vi "최치원저격용.vi"() -> ()   [LabVIEW 2015]
uses:
  <vilib>/NXT/Block Support/NXT_OutputPort.ctl
  <vilib>/NXT/Block Support/NXT_InputPort.ctl
  <vilib>/NXT/Subs/MotorOutput.ctl
  <vilib>/NXT/NXTIO Xnodes/NXTIONodeSubVIs/NXTMoveMotors.vi
  <vilib>/NXT/Dual Mode Library/Waits/Wait_Num.vi
  <vilib>/NXT/Dual Mode Library/Sensors/Sonar_cm.vi
  <vilib>/NXT/Dual Mode Library/Motors/MotorOn.vi
  <vilib>/NXT/Dual Mode Library/Waits/Wait_Rotation.vi
  <vilib>/NXT/Dual Mode Library/Sensors/Light_On.vi
  <vilib>/NXT/Dual Mode Library/Motors/MotorReverse.vi
  <vilib>/NXT/NXTIO Xnodes/AddressXNode/NXTIOAddress.xnode
  <vilib>/NXT/Subs/LVHSConnector.ctl
  <vilib>/NXT/NXTIO Xnodes/NXTIOXNode/NXTIO.xnode
  <vilib>/NXT/LegoClasses/BrickReference/BrickReference.lvclass
panel:
  in  "직진속도":i8=75
  in  "정지":bool
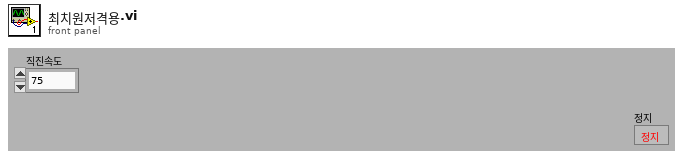
[diagram p1: front panel]
types:
  T1 = typedef "NXT_OutputPort.ctl" = u8
  T2 = typedef "LVHSConnector.ctl" = refnum<class "BrickReference.lvclass">
  T3 = typedef "MotorOutput.ctl" = u8
  T4 = typedef "NXT_InputPort.ctl" = u32
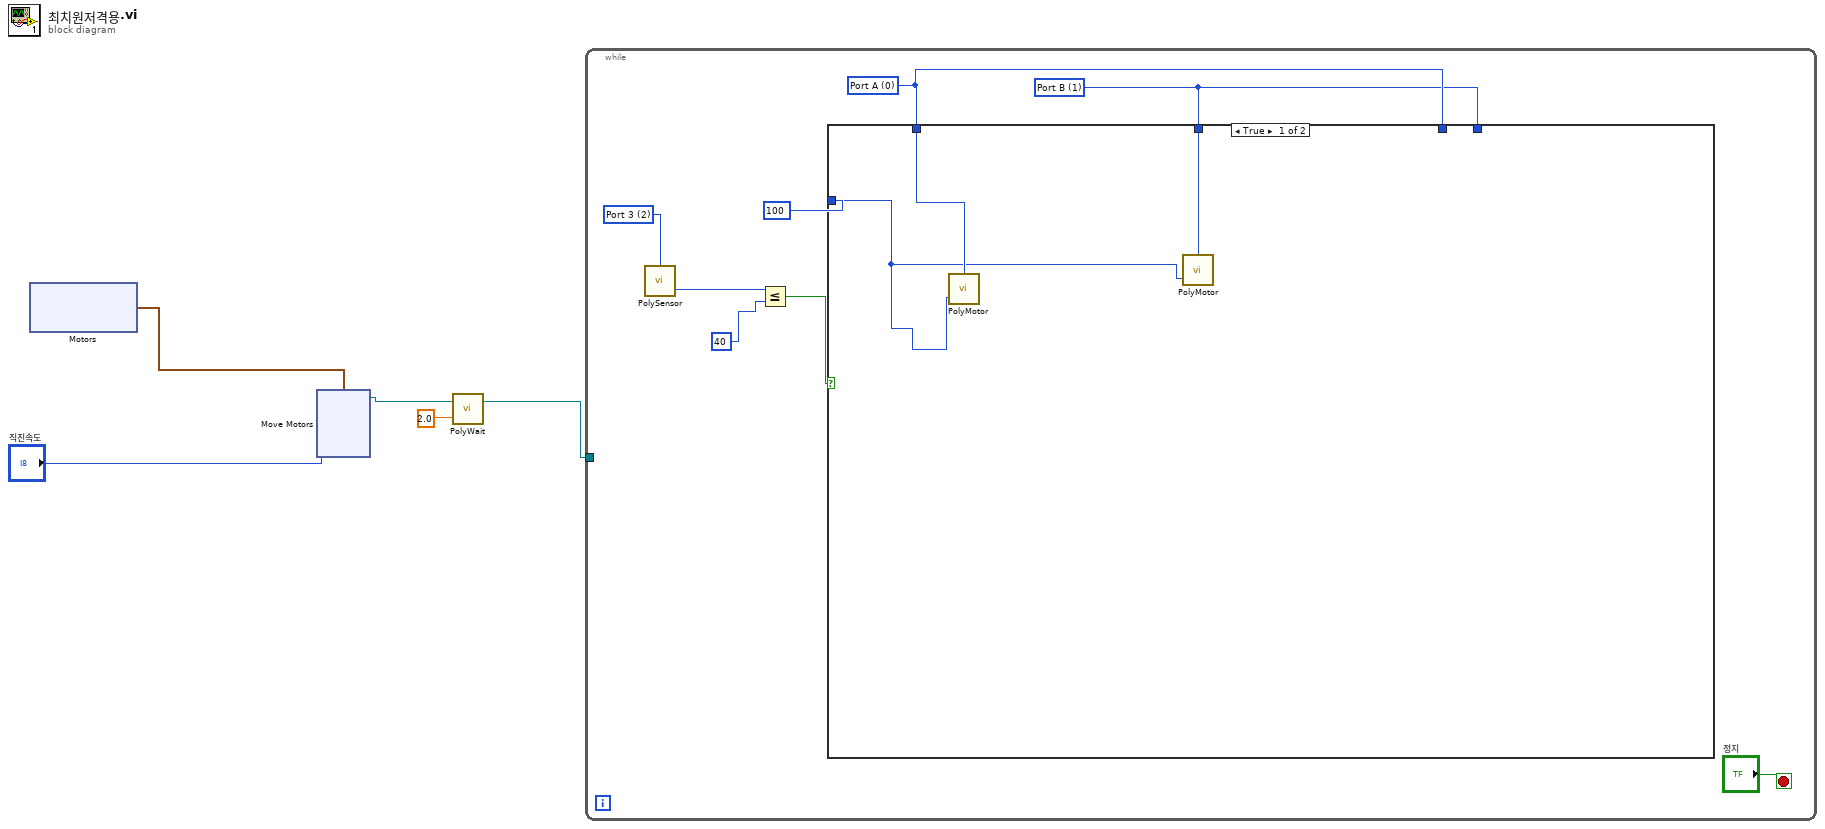
[diagram p0: block diagram]
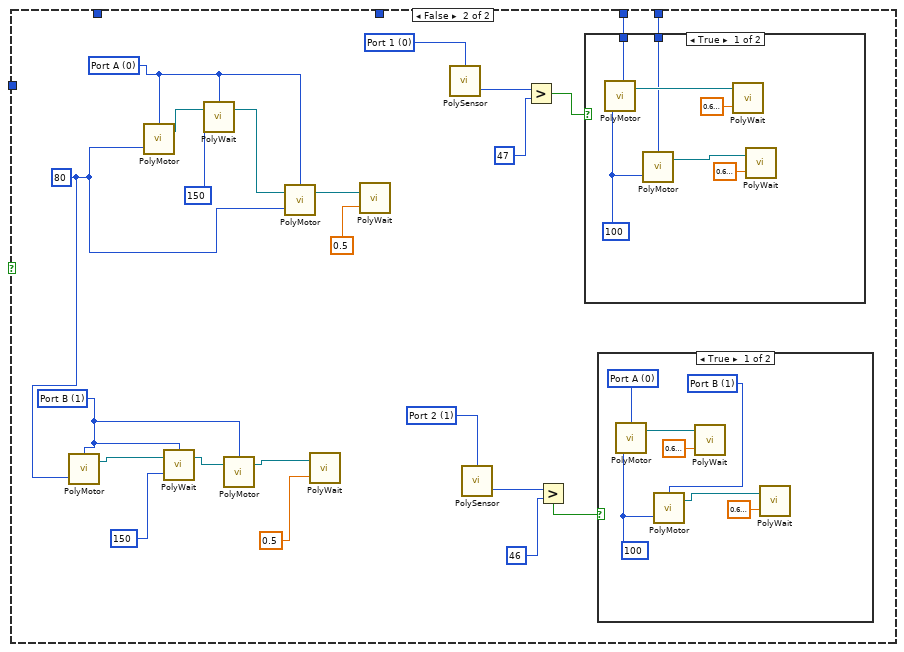
[diagram p2: hidden frame]
diagram:
  n1 = xnode "Motors"() -> ("Motor"=w5:cluster{"Port":T1, "Port":T1})
  n2 = xnode "Move Motors"("Power/Speed 1"="직진속도", "Motors"=w5, "Power/Speed 2"="직진속도") -> ("NXT/EV3"=w4:T2)  [unwired: 1 in]
  n3 = call-poly <vilib>:"PolyWait.vi"("Time (1 sec)"=sgl 2.0, "NXT/EV3"=w4) -> ("NXT/EV3"=w1:T2)  [unwired: 2 in]
  n4 = while {
    tunnel: w1 -> [_]
    stop <- "정지" stop-if-true
    w6 = T3 1 items=["Port A", "Port B", "Port C", "All Ports"] ("Output Port (All Ports)")
    w7 = T3 0 items=["Port A", "Port B", "Port C", "All Ports"] ("Output Port (All Ports)")
    w10 = T4 2 items=["Port 1", "Port 2", "Port 3", "Port 4"] ("Input Port")
    n5 = call-poly <vilib>:"PolySensor.vi"("Port (Port 4)"=w10) -> ("Distance (cm)"=w8:i16)  [unwired: 2 in, 1 out]
    n6 = Less Or Equal?(x=w8, y=40) -> (x <= y?=w11:bool)
    n7 = case shown="True" w11 {
      tunnel: w7 -> [w16 _]
      tunnel: 100 ("Power (75)") -> [w14 _]
      tunnel: w6 -> [w15 _]
      tunnel: w7 -> [_ w25]
      tunnel: w6 -> [_ w24]
      frame True {
        n8 = call-poly <vilib>:"PolyMotor.vi"("Power (75)"=w14, "Output Port (All Ports)"=w16) -> ()  [unwired: 2 in, 1 out]
        n9 = call-poly <vilib>:"PolyMotor.vi"("Power (75)"=w14, "Output Port (All Ports)"=w15) -> ()  [unwired: 2 in, 1 out]
      }
      frame False {
        w17 = T3 1 items=["Port A", "Port B", "Port C", "All Ports"] ("Output Port (All Ports)")
        w27 = T4 1 items=["Port 1", "Port 2", "Port 3", "Port 4"] ("Input Port")
        w26 = T4 0 items=["Port 1", "Port 2", "Port 3", "Port 4"] ("Input Port")
        w20 = 80 ("Power (75)")
        w34 = T3 0 items=["Port A", "Port B", "Port C", "All Ports"] ("Output Port (All Ports)")
        n10 = call-poly <vilib>:"PolyMotor.vi"("Power (75)"=w20, "Output Port (All Ports)"=w17) -> ("NXT/EV3"=w21:T2)  [unwired: 2 in]
        n11 = call-poly <vilib>:"PolyMotor.vi"("Power (75)"=w20, "Output Port (All Ports)"=w34) -> ("NXT/EV3"=w39:T2)  [unwired: 2 in]
        n12 = call-poly <vilib>:"PolyWait.vi"("Position Change (180)"=150, "NXT/EV3"=w21, "Port (Port A)"=w17) -> ("NXT/EV3"=w22:T2)  [unwired: 1 in]
        n13 = call-poly <vilib>:"PolyWait.vi"("Position Change (180)"=150, "NXT/EV3"=w39, "Port (Port A)"=w34) -> ("NXT/EV3"=w37:T2)  [unwired: 1 in]
        n14 = call-poly <vilib>:"PolyMotor.vi"("NXT/EV3"=w22, "Output Port (All Ports)"=w17) -> ("NXT/EV3"=w23:T2)  [unwired: 2 in]
        n15 = call-poly <vilib>:"PolyMotor.vi"("Power (75)"=w20, "NXT/EV3"=w37, "Output Port (All Ports)"=w34) -> ("NXT/EV3"=w36:T2)  [unwired: 1 in]
        n16 = call-poly <vilib>:"PolyWait.vi"("Time (1 sec)"=sgl 0.5, "NXT/EV3"=w23) -> ()  [unwired: 2 in, 1 out]
        n17 = call-poly <vilib>:"PolyWait.vi"("Time (1 sec)"=sgl 0.5, "NXT/EV3"=w36) -> ()  [unwired: 2 in, 1 out]
        n18 = call-poly <vilib>:"PolySensor.vi"("Port (Port 3)"=w26) -> ("Scaled Value"=w30:i16)  [unwired: 2 in, 1 out]
        n19 = call-poly <vilib>:"PolySensor.vi"("Port (Port 3)"=w27) -> ("Scaled Value"=w33:i16)  [unwired: 2 in, 1 out]
        n20 = Greater?(x=w30, y=47) -> (0:w28:bool)
        n21 = Greater?(x=w33, y=46) -> (0:w31:bool)
        n22 = case shown="True" w28 {
          tunnel: w25 -> [w44 _]
          tunnel: w24 -> [w41 _]
          frame True {
            w40 = 100 ("Power (75)")
            n23 = call-poly <vilib>:"PolyMotor.vi"("Power (75)"=w40, "Output Port (All Ports)"=w44) -> ("NXT/EV3"=w46:T2)  [unwired: 2 in]
            n24 = call-poly <vilib>:"PolyMotor.vi"("Power (75)"=w40, "Output Port (All Ports)"=w41) -> ("NXT/EV3"=w42:T2)  [unwired: 2 in]
            n25 = call-poly <vilib>:"PolyWait.vi"("Time (1 sec)"=sgl 0.7 ("Time (sec)"), "NXT/EV3"=w46) -> ()  [unwired: 2 in, 1 out]
            n26 = call-poly <vilib>:"PolyWait.vi"("Time (1 sec)"=sgl 0.7 ("Time (sec)"), "NXT/EV3"=w42) -> ()  [unwired: 2 in, 1 out]
          }
          frame False {
          }
        }
        n27 = case shown="True" w31 {
          frame True {
            w48 = T3 1 items=["Port A", "Port B", "Port C", "All Ports"] ("Output Port (All Ports)")
            w51 = T3 0 items=["Port A", "Port B", "Port C", "All Ports"] ("Output Port (All Ports)")
            w47 = 100 ("Power (75)")
            n28 = call-poly <vilib>:"PolyMotor.vi"("Power (75)"=w47, "Output Port (All Ports)"=w51) -> ("NXT/EV3"=w53:T2)  [unwired: 2 in]
            n29 = call-poly <vilib>:"PolyMotor.vi"("Power (75)"=w47, "Output Port (All Ports)"=w48) -> ("NXT/EV3"=w49:T2)  [unwired: 2 in]
            n30 = call-poly <vilib>:"PolyWait.vi"("Time (1 sec)"=sgl 0.7 ("Time (sec)"), "NXT/EV3"=w53) -> ()  [unwired: 2 in, 1 out]
            n31 = call-poly <vilib>:"PolyWait.vi"("Time (1 sec)"=sgl 0.7 ("Time (sec)"), "NXT/EV3"=w49) -> ()  [unwired: 2 in, 1 out]
          }
          frame False {
          }
        }
      }
    }
  }
